vi "Move group.vi"(0 "New handle position in":T1, 1 "Trap cluster in":T2, 2 "Previous handle position in":T1, 3 "Amplitudes":dbl[](array[numeric]), 4 "Group":bool[](array[boolean]), 5 "Switch X/Y":bool, 6 "Move handle":bool, 7 "Z":dbl[](array[numeric])) -> (8 "Trap cluster out":T2)   [LabVIEW 2009]
uses:
  Trap cluster.ctl
  <vilib>/Analysis/coordinate.llb/2D Cartesian Coordinate Shift (Array).vi
  <vilib>/Analysis/coordinate.llb/2D Cartesian Coordinate Rotation (Scalar).vi
  <vilib>/Analysis/NI_AALPro.lvlib
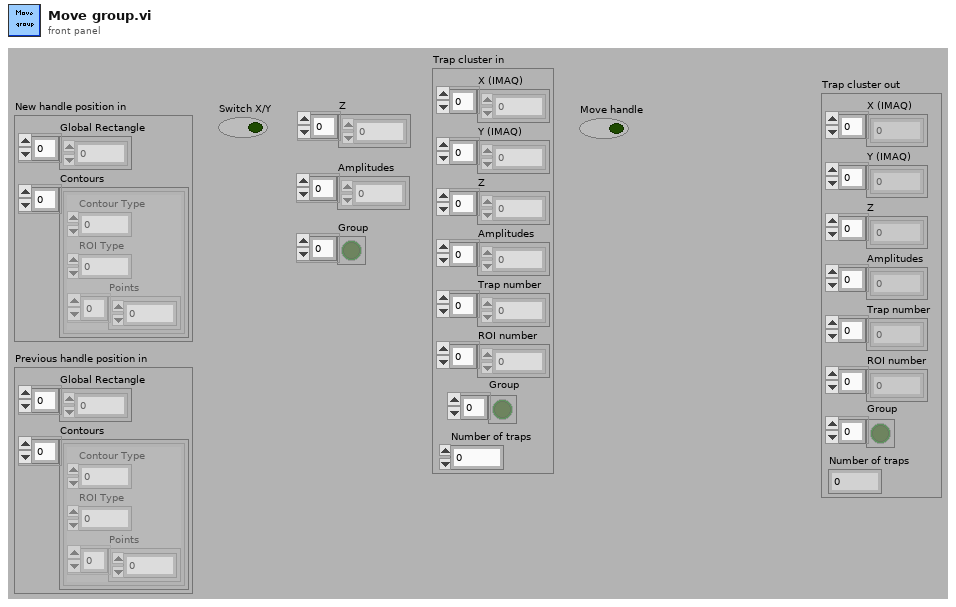
[diagram p1: front panel]
types:
  T1 = cluster{"Global Rectangle":i32[], "Contours":cluster{"Contour Type":u32, "ROI Type":u32, "Points":i32[]}[]}
  T2 = typedef "Trap cluster.ctl" = cluster{"X (IMAQ)":dbl[], "Y (IMAQ)":dbl[], "Z":dbl[], "Amplitudes":dbl[], "Trap number":i32[], "ROI number":i32[], "Number of traps":i32, "Group":bool[]}
  T3 = cluster{"Contour Type":u32, "ROI Type":u32, "Points":i32[]}[]
  T4 = cluster{"Contour Type":u32, "ROI Type":u32, "Points":i32[]}
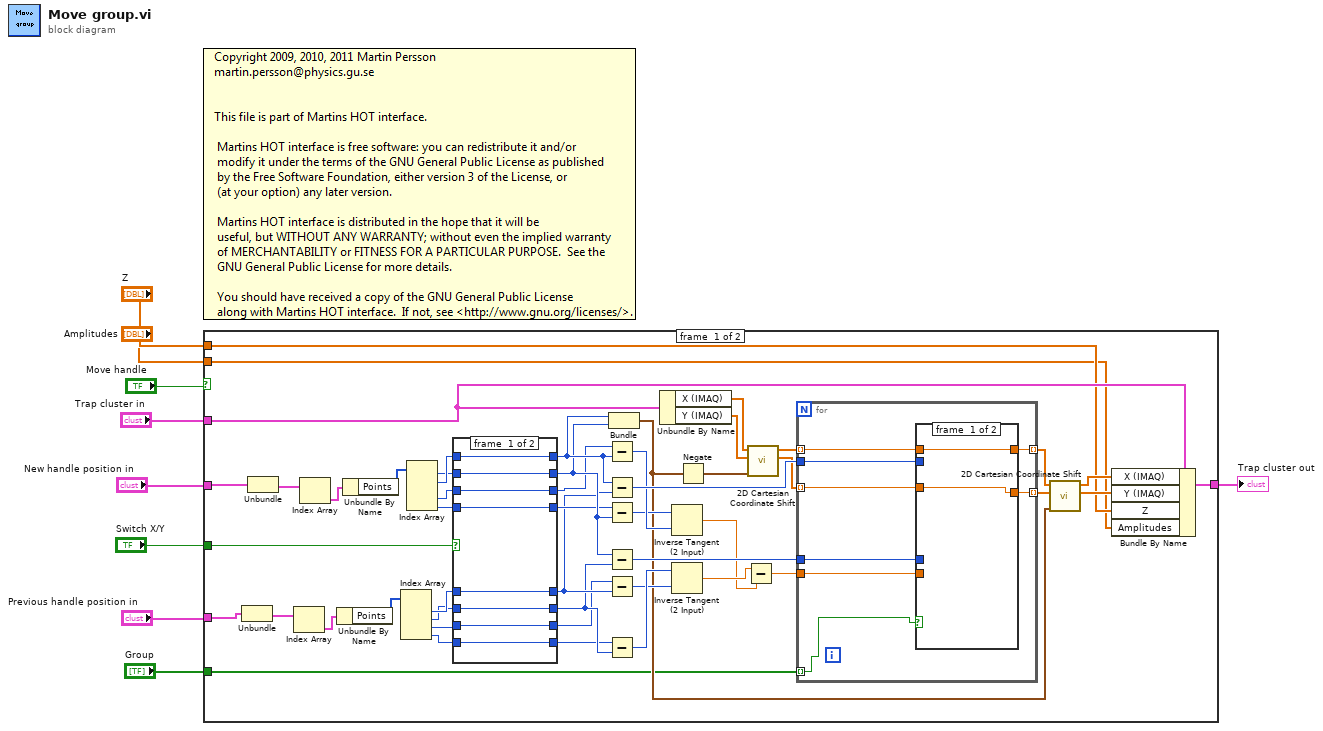
[diagram p0: block diagram]
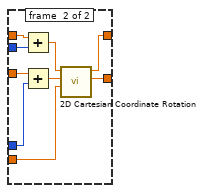
[diagram p3: hidden frame]
diagram:
  n1 = case shown="False" "Move handle" {
    tunnel: "Previous handle position in" -> [w11 _]
    tunnel: "Trap cluster in" -> [w58 w94]
    tunnel: [w57 w94] -> w7
    tunnel: "New handle position in" -> [w19 _]
    tunnel: "Z" -> [w37 _]
    tunnel: "Switch X/Y" -> [w28 _]
    tunnel: "Amplitudes" -> [w27 _]
    tunnel: "Group" -> [w10 _]
    frame #0 {
      n2 = Unbundle(w11) -> ("Contours"=w16:T3)  [unwired: 1 out]
      n3 = Unbundle(w19) -> ("Contours"=w26:T3)  [unwired: 1 out]
      n4 = Index Array(array=w16) -> (element=w17:T4)  [unwired: 1 in]
      n5 = Index Array(array=w26) -> (element=w25:T4)  [unwired: 1 in]
      n6 = Unbundle By Name(w17) -> ("Points"=w18:i32[])
      n7 = Unbundle By Name(w25) -> ("Points"=w24:i32[])
      n8 = Index Array(array=w18) -> (element #1=w13:i32, element #2=w12:i32, element #3=w15:i32, element #4=w14:i32)  [unwired: 4 in]
      n9 = Index Array(array=w24) -> (element #1=w23:i32, element #2=w22:i32, element #3=w21:i32, element #4=w20:i32)  [unwired: 4 in]
      n10 = case shown="True" w28 {
        tunnel: w23 -> [w66 w74]
        tunnel: [w66 w73] -> w36
        tunnel: w22 -> [w65 w73]
        tunnel: [w65 w74] -> w35
        tunnel: w21 -> [w64 w72]
        tunnel: [w64 w71] -> w34
        tunnel: w20 -> [w63 w71]
        tunnel: [w63 w72] -> w33
        tunnel: w13 -> [w62 w70]
        tunnel: [w62 w69] -> w32
        tunnel: w12 -> [w61 w69]
        tunnel: [w61 w70] -> w31
        tunnel: w15 -> [w60 w68]
        tunnel: [w60 w67] -> w30
        tunnel: w14 -> [w59 w67]
        tunnel: [w59 w68] -> w29
        frame #0 {
        }
        frame #1 {
        }
      }
      n11 = Subtract(x=w34, y=w36) -> (x-y=w54:i32)
      n12 = Subtract(x=w36, y=w32) -> (x-y=w56:i32)
      n13 = Subtract(x=w33, y=w35) -> (x-y=w53:i32)
      n14 = Subtract(x=w35, y=w31) -> (x-y=w55:i32)
      n15 = Subtract(x=w30, y=w32) -> (x-y=w51:i32)
      n16 = Subtract(x=w29, y=w31) -> (x-y=w52:i32)
      n17 = Bundle(w36, w35) -> (w43:cluster{i32, i32})  [unwired: 1 in]
      n18 = Unbundle By Name(w58) -> ("X (IMAQ)"=w50:dbl[], "Y (IMAQ)"=w49:dbl[])
      n19 = Inverse Tangent (2 Input)(1:w54, 2:w53) -> (0:w38:dbl)
      n20 = Inverse Tangent (2 Input)(1:w51, 2:w52) -> (0:w39:dbl)
      n21 = Negate(x=w43) -> (-x=w42:cluster{i32, i32})
      n22 = Subtract(x=w39, y=w38) -> (x-y=w46:dbl)
      n23 = call-poly <vilib>:"2D Cartesian Coordinate Shift.vi"("shift"=w42, "Y"=w49, "X"=w50) -> ("Y Out"=w47:dbl[], "X Out"=w48:dbl[])  [unwired: 6 in, 1 out]
      n24 = for {
        tunnel: w48 -> [w82] mode=indexing
        tunnel: w47 -> [w81] mode=indexing
        tunnel: w56 -> [w80]
        tunnel: w55 -> [w79]
        tunnel: [w78] -> w45 mode=indexing
        tunnel: [w77] -> w44 mode=indexing
        tunnel: w46 -> [w76]
        tunnel: w10 -> [w75] mode=indexing
        n25 = case shown="True" w75 {
          tunnel: w82 -> [w84 w93]
          tunnel: w81 -> [w83 w91]
          tunnel: w80 -> [_ w92]
          tunnel: w79 -> [_ w90]
          tunnel: [w84 w86] -> w78
          tunnel: [w83 w85] -> w77
          tunnel: w76 -> [_ w87]
          frame #0 {
          }
          frame #1 {
            n26 = Add(x=w93, y=w92) -> (x+y=w89:dbl)
            n27 = Add(x=w91, y=w90) -> (x+y=w88:dbl)
            n28 = call-poly <vilib>:"2D Cartesian Coordinate Rotation.vi"("theta"=w87, "y"=w88, "x"=w89) -> ("y out"=w85:dbl, "x out"=w86:dbl)  [unwired: 6 in, 1 out]
          }
        }
      }
      n29 = call-poly <vilib>:"2D Cartesian Coordinate Shift.vi"("shift"=w43, "Y"=w44, "X"=w45) -> ("Y Out"=w40:dbl[], "X Out"=w41:dbl[])  [unwired: 6 in, 1 out]
      n30 = Bundle By Name(cluster=w58, "X (IMAQ)"=w41, "Y (IMAQ)"=w40, "Z"=w37, "Amplitudes"=w27) -> (w57:T2)
    }
    frame #1 {
    }
  }
  "Trap cluster out" <- w7
